vi "getpath.vi"() -> (3 "stripped path":path)   [LabVIEW 2013]
panel:
  out "Application Directory":path caption="应用程序目录"
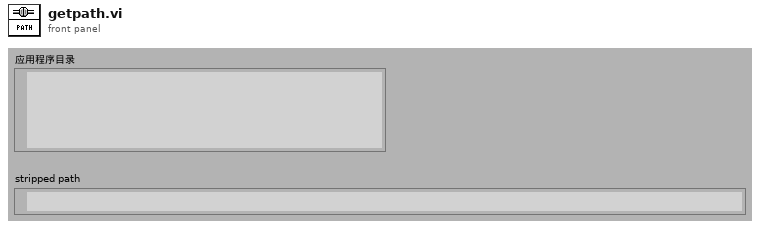
[diagram p1: front panel]
types:
  T1 = enum32{"invalid app kind", "Development System", "Run Time System", "Student Edition", "Embedded LabVIEW", "Evaluation", "Custom"}
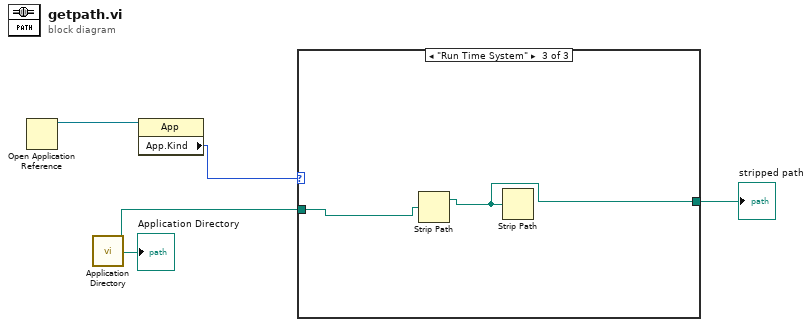
[diagram p0: block diagram]
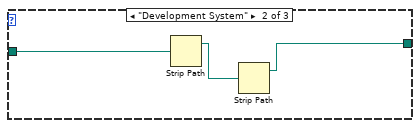
[diagram p3: hidden frame]
diagram:
  n1 = Open Application Reference() -> (3:w4:refnum<vi>)  [unwired: 1 in, 4 out]
  n2 = call <vilib>:"Application Directory.vi"() -> ("Application Directory"=w2:path)
  "Application Directory" <- w2
  n3 = property class="App"(reference=w4) -> ("App.Kind"=w3:T1)  [unwired: 1 in, 2 out]
  n4 = case shown="\"Run Time System\"" w3 {
    tunnel: w2 -> [w5 w8 w10]
    tunnel: [w5 w6 w9] -> w1
    frame "invalid app kind", Default {
    }
    frame "Development System" {
      n5 = Strip Path(path=w8) -> (stripped path=w7:path)  [unwired: 1 out]
      n6 = Strip Path(path=w7) -> (stripped path=w6:path)  [unwired: 1 out]
    }
    frame "Run Time System" {
      n7 = Strip Path(path=w10) -> (stripped path=w9:path)  [unwired: 1 out]
      n8 = Strip Path(path=w9) -> ()  [unwired: 2 out]
    }
  }
  "stripped path" <- w1
